vi "Enqueue ACQ Element.vi"(8 "error in (no error)":errorcluster, 10 "1 Sample":T1, 11 "ACQ Data Queue in":refnum<queue>) -> (0 "error out":errorcluster, 3 "ACQ Data Queue out":refnum<queue>)   [LabVIEW 2014, in "WINFAS 2 Data Queue.lvlib"]
uses:
  WINFAS 2 Data Queue.lvlib
  Acquisition Data 1 Sample Cluster.ctl
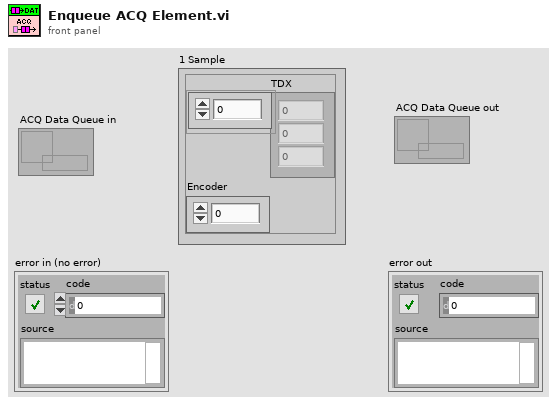
[diagram p1: front panel]
types:
  T1 = typedef "WINFAS 2 Data Queue.lvlib/Acquisition Data 1 Sample Cluster.ctl" = cluster{"TDX":sgl[], "Encoder":sgl}
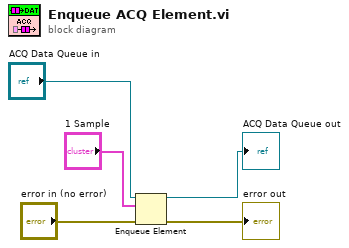
[diagram p0: block diagram]
diagram:
  n1 = Enqueue Element(queue="ACQ Data Queue in", element="1 Sample", error in (no error)="error in (no error)") -> (queue out=→"ACQ Data Queue out":refnum<queue>, error out=→"error out":errorcluster)  [unwired: 1 in, 1 out]
